vi "resolução.vi"() -> ()   [LabVIEW 2017]
uses:
  <vilib>/userdefined/High Color/IMAQdx.ctl
  <vilib>/vision/driver/IMAQdx.llb/IMAQdx Acquisition Mode.ctl
  <vilib>/vision/driver/IMAQdx.llb/IMAQdx Buffer Number Mode.ctl
  <vilib>/vision/driver/NI_Vision_Acquisition_Software.lvlib
  <vilib>/vision/NI_Vision_Development_Module.lvlib
panel:
  in  "Y Resolution":i32
  in  "X Resolution":i32
  out "Imagem Original 2":T1(plugin-control)
  out "error out":errorcluster
  out "Imagem Original":T1(plugin-control)
  in  "Stop Button":bool
  in  "Câmera":T2="cam1"
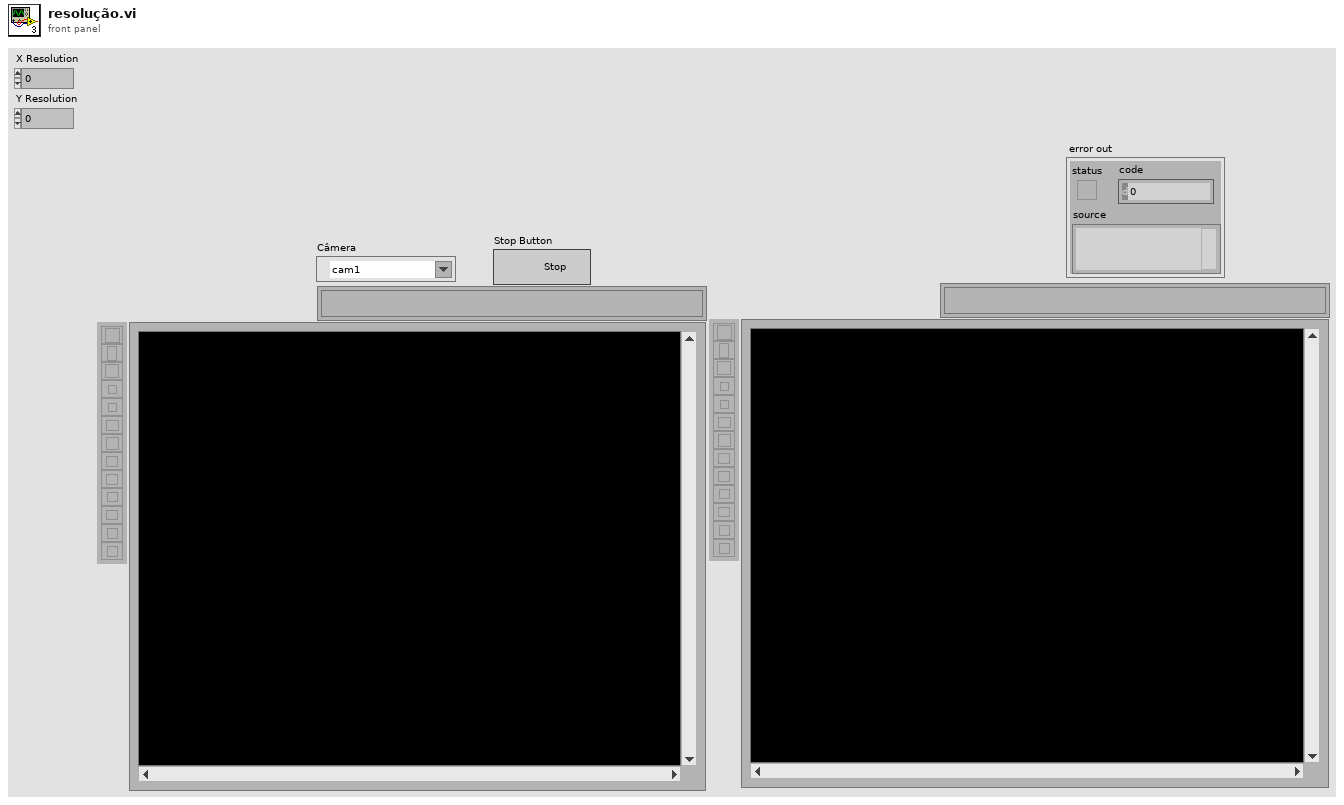
[diagram p1: front panel]
types:
  T1 = typedef "IMAQ Image.ctl" = refnum<image>
  T2 = typedef "IMAQdx.ctl" = refnum<k21>
  T3 = typedef "Image Type" = u32
  T4 = typedef "NI_Vision_Acquisition_Software.lvlib/IMAQdx Acquisition Mode.ctl" = enum32{"One Shot", "Continuous"}
  T5 = typedef "NI_Vision_Acquisition_Software.lvlib/IMAQdx Buffer Number Mode.ctl" = enum32{"Next", "Last", "Buffer Number", "Every", "Last New"}
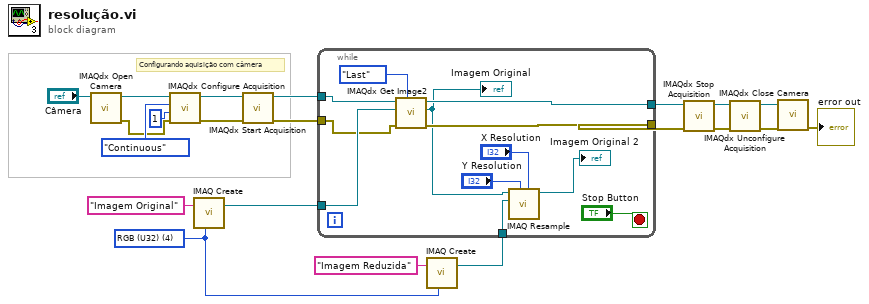
[diagram p0: block diagram]
diagram:
  w1 = T3 4 items=["Grayscale (U8)", "Grayscale (I16)", "Grayscale (SGL)", "Complex (CSG)", "RGB (U32)", "HSL (U32)", "RGB (U64)", "Grayscale (U16)"] ("Image Type")
  # "Configurando aquisição com câmera"
  n1 = call <vilib>:"IMAQdx Open Camera.vi"("Session In"="Câmera") -> ("error out"=w12:errorcluster, "Session Out"=w21:T2)  [unwired: 9 in]
  n2 = call <vilib>:"IMAQdx Configure Acquisition.vi"("error in"=w12, "Number of Buffers"=u32 1, "Continuous?"=IMAQdx_Acquisition_Mode."Continuous", "Session In"=w21) -> ("error out"=w13:errorcluster, "Session Out"=w20:T2)  [unwired: 6 in]
  n3 = call "IMAQ Create"("Image Name"="Imagem Original", "Image Type"=w1) -> ("New Image"=w7:T1)  [unwired: 3 in, 1 out]
  n4 = call <vilib>:"IMAQdx Start Acquisition.vi"("error in"=w13, "Session In"=w20) -> ("error out"=w14:errorcluster, "Session Out"=w15:T2)  [unwired: 8 in]
  n5 = call "IMAQ Create"("Image Name"="Imagem Reduzida", "Image Type"=w1) -> ("New Image"=w2:T1)  [unwired: 3 in, 1 out]
  n6 = while {
    tunnel: w15 -> [w28]
    tunnel: w14 -> [w27]
    tunnel: [w31] -> w9
    tunnel: [w30] -> w8
    tunnel: w7 -> [w29]
    tunnel: w2 -> [w23]
    stop <- "Stop Button" stop-if-true
    n7 = call <vilib>:"IMAQdx Get Image2.vi"("Buffer Number Mode (Next)"=IMAQdx_Buffer_Number_Mode."Last", "error in"=w27, "Image In"=w29, "Session In"=w28) -> ("error out"=w30:errorcluster, "Image Out"=w24:T1, "Session Out"=w31:T2)  [unwired: 4 in, 1 out]
    "Imagem Original" <- w24
    n8 = call "IMAQ Resample"("X Resolution"="X Resolution", "Y Resolution"="Y Resolution", "Image Dst"=w23, "Image Src"=w24) -> ("Image Dst Out"=→"Imagem Original 2":T1)  [unwired: 6 in, 1 out]
  }
  n9 = call <vilib>:"IMAQdx Stop Acquisition.vi"("error in"=w8, "Session In"=w9) -> ("error out"=w6:errorcluster, "Session Out"=w11:T2)  [unwired: 8 in]
  n10 = call <vilib>:"IMAQdx Unconfigure Acquisition.vi"("error in"=w6, "Session In"=w11) -> ("error out"=w5:errorcluster, "Session Out"=w10:T2)  [unwired: 8 in]
  n11 = call <vilib>:"IMAQdx Close Camera.vi"("error in"=w5, "Session In"=w10) -> ("error out"=→"error out":errorcluster)  [unwired: 9 in]
